vi "Pause Message.vi"(3 "字符串":string, 4 "SEQ":i32, 5 "tpdata":string[](array[string])) -> (2 "ta data out":string[](array[string]))   [LabVIEW 2018]
panel:
  in  "Cancel":bool
  in  "OK":bool
  in  "备注":string
  in  "Output string":string
  # "提示信息设置"
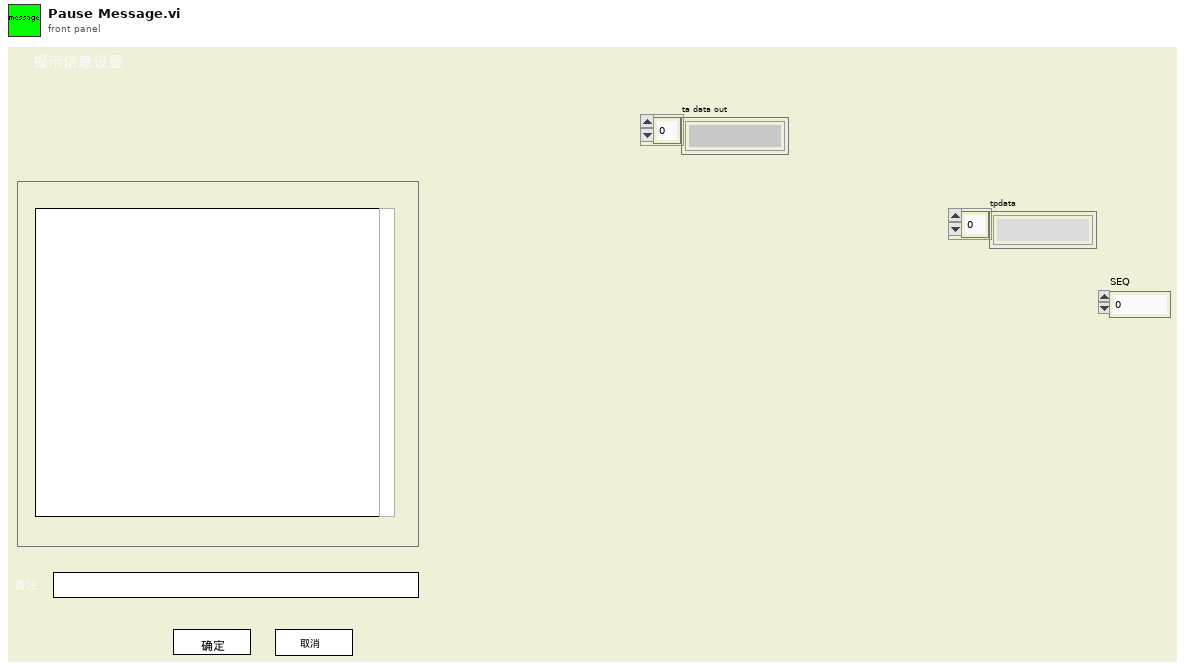
[diagram p1: front panel]
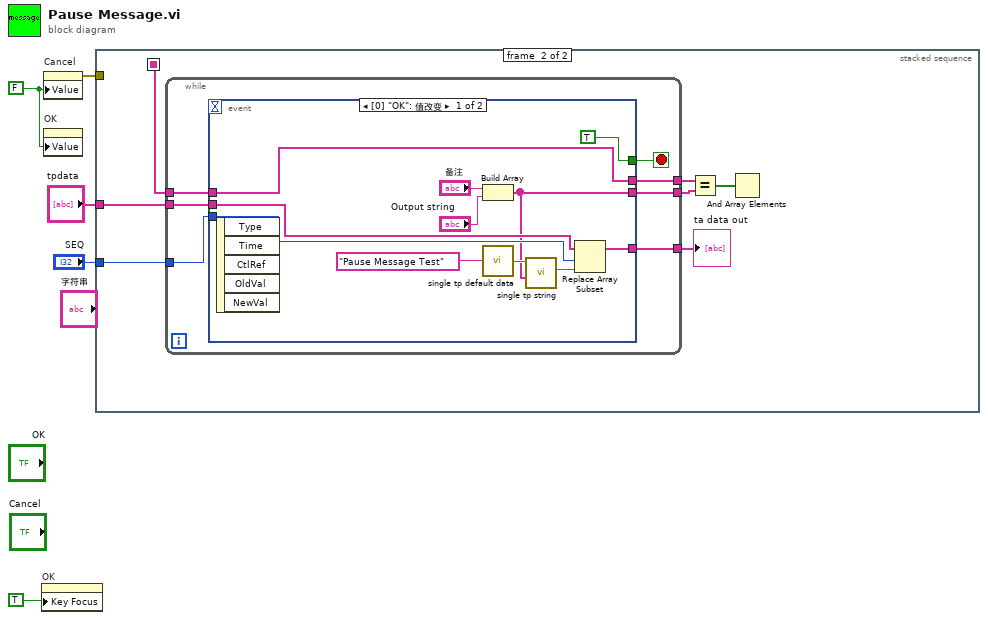
[diagram p0: block diagram]
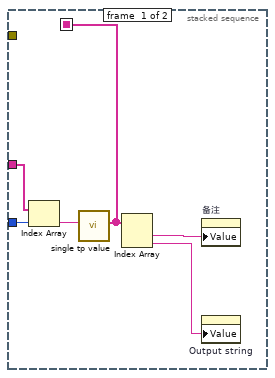
[diagram p2: hidden frame]
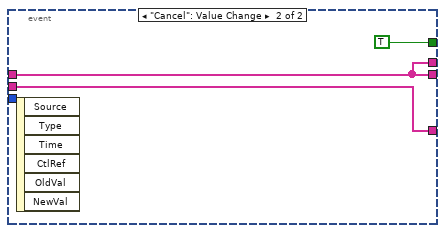
[diagram p3: hidden frame]
diagram:
  w4 = FALSE
  n1 = property on="OK" class="Bool (严格)"("Key Focus"=TRUE) -> ()  [unwired: 2 in, 2 out]
  n2 = property on="Cancel" class="Bool (严格)"("Value"=w4) -> (error out=w5:errorcluster)  [unwired: 2 in, 1 out]
  n3 = property on="OK" class="Bool (严格)"("Value"=w4) -> ()  [unwired: 2 in, 2 out]
  n4 = stacked-sequence {
    seq-local: [w6 _] -> [_ w16]
    tunnel: "SEQ" -> [w9 w17]
    tunnel: w5 -> [_ _]
    tunnel: "tpdata" -> [w10 w18]
    frame #0 {
      n5 = Index Array(array=w10, index=w9) -> (element=w8:string)
      n6 = call "single tp value.vi"("single tp data"=w8) -> ("value"=w6:string[])  [unwired: 10 out]
      n7 = Index Array(array=w6) -> (element #1=w7:string, element #2=w11:string)  [unwired: 2 in]
      n8 = property on="备注" class="Str"("Value"=w7) -> ()  [unwired: 2 in, 2 out]
      n9 = property on="Output string" class="Str"("Value"=w11) -> ()  [unwired: 2 in, 2 out]
    }
    frame #1 {
      n10 = while {
        tunnel: w18 -> [w24]
        tunnel: w17 -> [w23]
        tunnel: [w22] -> w15
        tunnel: [w21] -> w12
        tunnel: w16 -> [w20]
        tunnel: [w19] -> w13
        stop <- w25 stop-if-true
        n11 = event shown="[0] \"OK\": 值改变" {
          selector: _ -> [_ _]
          dyn-events: _ -> [_ _]
          timeout: _ -> [_ _]
          tunnel: [TRUE TRUE] -> w25
          tunnel: w24 -> [w31 w38]
          tunnel: w23 -> [w30 _]
          tunnel: [w28 w38] -> w22
          tunnel: [w27 w37] -> w21
          tunnel: w20 -> [w26 w37]
          tunnel: [w26 w37] -> w19
          event "OK": Value Change {
            n12 = event-data() -> ()  [unwired: 6 out]
            n13 = Build Array("备注", "Output string") -> (w27:string[])
            n14 = call "single tp default data.vi"("字符串"="Pause Message Test" ("test item")) -> ("item data"=w32:string)
            n15 = call "single tp string.vi"("value in"=w27, "oringnal defult tp data"=w32) -> ("new single tp data out"=w29:string)  [unwired: 9 out]
            n16 = Replace Array Subset(array=w31, new element=w29, index=w30) -> (w28:string[])
          }
          event "Cancel": Value Change {
            n17 = event-data() -> ()  [unwired: 7 out]
          }
        }
      }
      "ta data out" <- w15
      n18 = Equal?(x=w13, y=w12) -> (x = y?=w14:bool[])
      n19 = And Array Elements(Boolean array=w14) -> ()  [unwired: 1 out]
    }
  }
